vi "10-1.vi"() -> ()   [LabVIEW 2022 SP3, in "AoC22.lvlib"]
uses:
  AoC22.lvlib
  <vilib>/IlluminatedG/lv-stream/Stream.lvlib
panel:
  out "Array 3":i32[](array[numeric])
  out "Array 2":i32[](array[numeric])
  out "Array":i32[](array[numeric])
  out "x < 0?":bool
  out "sum":i32
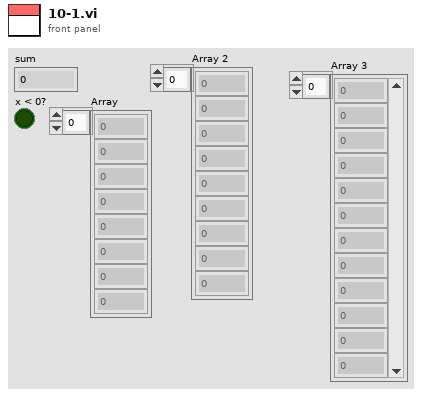
[diagram p1: front panel]
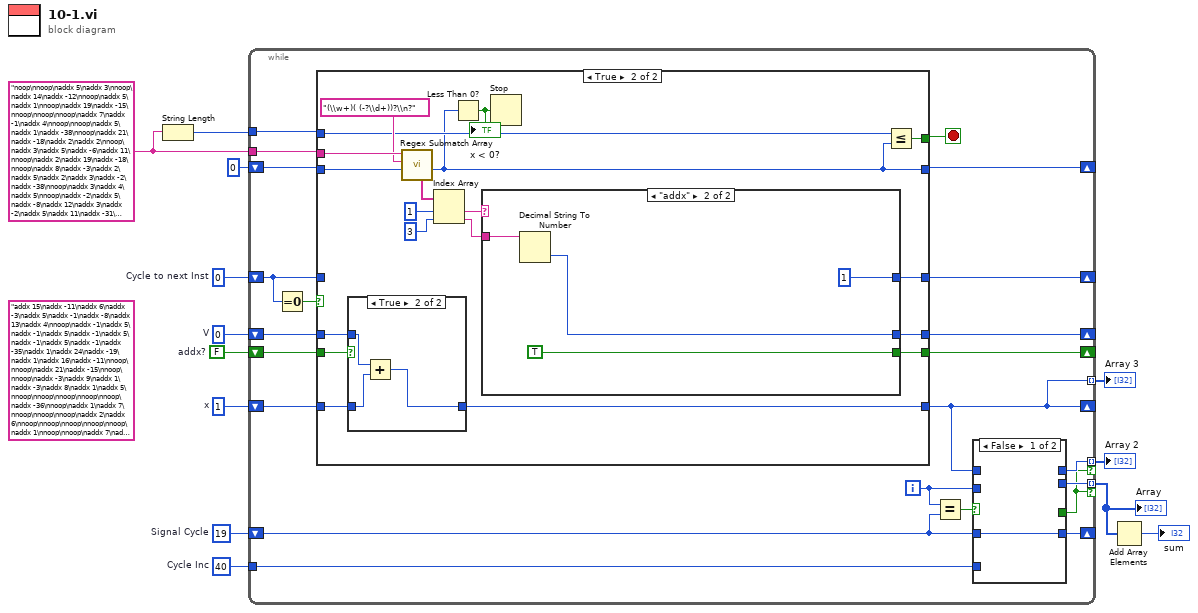
[diagram p0: block diagram]
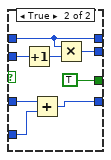
[diagram p2: hidden frame]
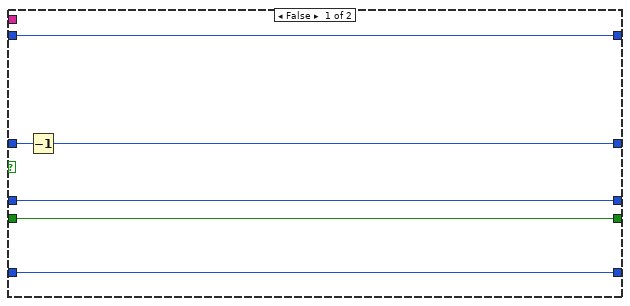
[diagram p3: hidden frame]
diagram:
  (unwired) "addx 15\naddx -11\naddx 6\naddx -3\naddx 5\naddx -1\naddx -8\naddx 13\naddx 4\nnoop\naddx -1\naddx 5\naddx -1\naddx 5\naddx -1\naddx 5\naddx -1\naddx 5\naddx -1\naddx -35\naddx 1\naddx 24\naddx -19\naddx 1\naddx 16\naddx -11\nnoop\nnoop\naddx 21\naddx -15\nnoop\nnoop\naddx -3\naddx 9\naddx 1\naddx -3\naddx 8\naddx 1\naddx 5\nnoop\nnoop\nnoop\nnoop\nnoop\naddx -36\nnoop\naddx 1\naddx 7\nnoop\nnoop\nnoop\naddx 2\naddx 6\nnoop\nnoop\nnoop\nnoop\nnoop\naddx 1\nnoop\nnoop\naddx 7\naddx 1\nnoop\naddx -13\naddx 13\naddx 7\nnoop\naddx 1\naddx -33\nnoop\nnoop\nnoop\naddx 2\nnoop\nnoop\nnoop\naddx 8\nnoop\naddx -1\naddx 2\naddx 1\nnoop\naddx 17\naddx -9\naddx 1\naddx 1\naddx -3\naddx 11\nnoop\nnoop\naddx 1\nnoop\naddx 1\nnoop\nnoop\naddx -13\naddx -19\naddx 1\naddx 3\naddx 26\naddx -30\naddx 12\naddx -1\naddx 3\naddx 1\nnoop\nnoop\nnoop\naddx -9\naddx 18\naddx 1\naddx 2\nnoop\nnoop\naddx 9\nnoop\nnoop\nnoop\naddx -1\naddx 2\naddx -37\naddx 1\naddx 3\nnoop\naddx 15\naddx -21\naddx 22\naddx -6\naddx 1\nnoop\naddx 2\naddx 1\nnoop\naddx -10\nnoop\nnoop\naddx 20\naddx 1\naddx 2\naddx 2\naddx -6\naddx -11\nnoop\nnoop\nnoop"
  w7 = 40  # Cycle Inc
  w8 = 19  # Signal Cycle
  w9 = FALSE  # addx?
  w11 = 1  # x
  w10 = 0  # V
  w12 = 0  # Cycle to next Inst
  w1 = "noop\nnoop\naddx 5\naddx 3\nnoop\naddx 14\naddx -12\nnoop\naddx 5\naddx 1\nnoop\naddx 19\naddx -15\nnoop\nnoop\nnoop\naddx 7\naddx -1\naddx 4\nnoop\nnoop\naddx 5\naddx 1\naddx -38\nnoop\naddx 21\naddx -18\naddx 2\naddx 2\nnoop\naddx 3\naddx 5\naddx -6\naddx 11\nnoop\naddx 2\naddx 19\naddx -18\nnoop\naddx 8\naddx -3\naddx 2\naddx 5\naddx 2\naddx 3\naddx -2\naddx -38\nnoop\naddx 3\naddx 4\naddx 5\nnoop\naddx -2\naddx 5\naddx -8\naddx 12\naddx 3\naddx -2\naddx 5\naddx 11\naddx -31\naddx 23\naddx 4\nnoop\nnoop\naddx 5\naddx 3\naddx -2\naddx -37\naddx 1\naddx 5\naddx 2\naddx 12\naddx -10\naddx 3\naddx 4\naddx -2\nnoop\naddx 6\naddx 1\nnoop\nnoop\nnoop\naddx -2\naddx 7\naddx 2\nnoop\naddx 3\naddx 3\naddx 1\nnoop\naddx -37\naddx 2\naddx 5\naddx 2\naddx 32\naddx -31\naddx 5\naddx 2\naddx 9\naddx 9\naddx -15\nnoop\naddx 3\naddx 2\naddx 5\naddx 2\naddx 3\naddx -2\naddx 2\naddx 2\naddx -37\naddx 5\naddx -2\naddx 2\naddx 5\naddx 2\naddx 16\naddx -15\naddx 4\nnoop\naddx 1\naddx 2\nnoop\naddx 3\naddx 5\naddx -1\naddx 5\nnoop\nnoop\nnoop\nnoop\naddx 3\naddx 5\naddx -16\nnoop"
  n1 = String Length(string=w1) -> (length=w13:i32)
  n2 = while {
    tunnel: w1 -> [w35]
    shift-right: [w32] -> _
    shift-left: 0 ("offset past match") -> [w34]
    tunnel: w13 -> [w33]
    shift-right: [w25] -> _
    shift-left: w12 -> [w29]
    shift-right: [w14] -> _
    shift-left: w11 -> [w27]
    shift-right: [w20] -> _
    shift-left: w10 -> [w28]
    shift-right: [w19] -> _
    shift-left: w9 -> [w26]
    shift-right: [w22] -> _
    shift-left: w8 -> [w23]
    tunnel: w7 -> [w21]
    tunnel: [w17] -> w6 mode=indexing if=w15
    tunnel: [w16] -> w3 mode=indexing if=w15
    tunnel: [w14] -> w2 mode=indexing
    i -> [w18]
    stop <- w31 stop-if-true
    n3 = Equal To 0?(x=w29) -> (x = 0?=w30:bool)
    n4 = case shown="True" w30 {
      tunnel: w35 -> [_ w69]
      tunnel: w34 -> [w45 w67]
      tunnel: w33 -> [_ w66]
      tunnel: [w45 w52] -> w32
      tunnel: [_ w65] -> w31
      tunnel: w29 -> [w50 _]
      tunnel: w28 -> [w47 w57]
      tunnel: w27 -> [w48 w58]
      tunnel: w26 -> [w46 w59]
      tunnel: [w49 w53] -> w25
      tunnel: [w48 w56] -> w14
      tunnel: [w47 w55] -> w20
      tunnel: [w46 w54] -> w19
      frame False {
        n5 = Decrement(x=w50) -> (x-1=w49:i32)
      }
      frame True {
        n6 = case shown="True" w59 {
          tunnel: w58 -> [w70 w73]
          tunnel: w57 -> [_ w72]
          tunnel: [w70 w71] -> w56
          frame False {
          }
          frame True {
            n7 = Add(x=w72, y=w73) -> (x+y=w71:i32)
          }
        }
        n8 = call <vilib>:"Regex Submatch Array.vi"("offset (0)"=w67, "regular expression"="(\\w+)( (-?\\d+))?\\n?", "string"=w69) -> ("offset past match"=w52:i32, "matches"=w64:string[])  [unwired: 6 in, 1 out]
        n9 = Index Array(array=w64, index #1=1 ("index"), index #2=3 ("index")) -> (element #1=w61:string, element #2=w60:string)
        n10 = Less Than 0?(x=w52) -> (x < 0?=w51:bool)
        "x < 0?" <- w51
        n11 = case shown="\"addx\"" w61 {
          tunnel: w60 -> [_ w77]
          tunnel: [_ w76] -> w55
          tunnel: [_ TRUE] -> w54
          tunnel: [_ 1] -> w53
          frame "noop", Default {
          }
          frame "addx" {
            n12 = Decimal String To Number(string=w77) -> (number=w76:i32)  [unwired: 2 in, 1 out]
          }
        }
        n13 = Stop(stop? (T)=w51) -> ()
        n14 = Less Or Equal?(x=w66, y=w52) -> (x <= y?=w65:bool)
      }
    }
    n15 = Equal?(x=w18, y=w23) -> (x = y?=w24:bool)
    n16 = case shown="False" w24 {
      tunnel: w23 -> [w36 w44]
      tunnel: [w36 w42] -> w22
      tunnel: w21 -> [_ w43]
      tunnel: w14 -> [_ w37]
      tunnel: w18 -> [_ w41]
      tunnel: [_ w39] -> w17
      tunnel: [_ TRUE] -> w15
      tunnel: [_ w37] -> w16
      frame False {
      }
      frame True {
        n17 = Increment(x=w41) -> (x+1=w40:i32)
        n18 = Add(x=w44, y=w43) -> (x+y=w42:i32)
        n19 = Multiply(x=w37, y=w40) -> (x*y=w39:i32)
      }
    }
  }
  "Array" <- w6
  "Array 2" <- w3
  "Array 3" <- w2
  n20 = Add Array Elements(numeric array=w6) -> (sum=→"sum":i32)
